vi "OnGameEnd.vi"(8 "error in (no error)":errorcluster, 11 "Game in":refnum<class "Game.lvclass">) -> (0 "error out":errorcluster, 3 "Game out":refnum<class "Game.lvclass">)   [LabVIEW 2019, in "RT_Game.lvlib" / "Game.lvclass"]
uses:
  Game.lvclass
  Game.lvclass/Game.ctl
  Menu/States.ctl
  Highscore/Highscore.lvclass
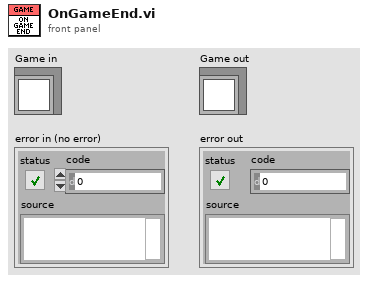
[diagram p1: front panel]
types:
  T1 = typedef "RT_Game.lvlib/Game.lvclass/States.ctl" = enum16{"Init", "Restart", "Menu", "Game", "Resume", "ToggleSingleplayer", "LoadNextGame", "ExitToMenu", "NewHighscore", "GameOver", "SlideOut"}
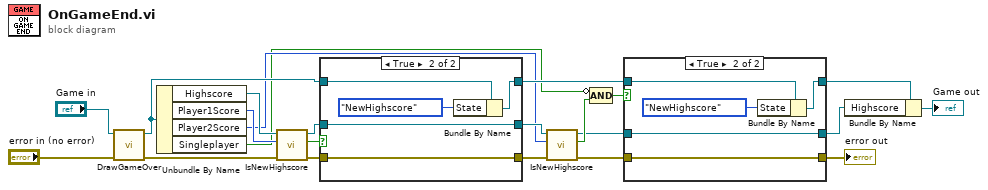
[diagram p0: block diagram]
diagram:
  n1 = call "DrawGameOver.vi"("error in (no error)"="error in (no error)", "Game in"="Game in") -> ("error out"=w20:errorcluster, "Game out"=w13:refnum<class "Game.lvclass">)  [unwired: 8 in]
  n2 = Unbundle By Name(w13) -> ("Highscore"=w18:refnum<class "Highscore.lvclass">, "Player1Score"=w17:i32, "Player2Score"=w6:i32, "Singleplayer"=w1:bool)
  n3 = call "IsNewHighscore.vi"("error in (no error)"=w20, "Score"=w17, "Highscore in"=w18) -> ("error out"=w16:errorcluster, "IsNewHighscore?"=w14:bool, "Highscore out"=w15:refnum<class "Highscore.lvclass">)  [unwired: 6 in]
  n4 = case shown="True" w14 {
    tunnel: w16 -> [w23 w30]
    tunnel: [w23 w30] -> w12
    tunnel: w15 -> [w24 w29]
    tunnel: [w24 w29] -> w11
    tunnel: w13 -> [w25 w28]
    tunnel: [w25 w27] -> w7
    frame False {
    }
    frame True {
      n5 = Bundle By Name(cluster=w28, "State"=States."NewHighscore") -> (w27:refnum<class "Game.lvclass">)
    }
  }
  n6 = call "IsNewHighscore.vi"("error in (no error)"=w12, "Score"=w6, "Highscore in"=w11) -> ("error out"=w3:errorcluster, "IsNewHighscore?"=w5:bool, "Highscore out"=w4:refnum<class "Highscore.lvclass">)  [unwired: 6 in]
  n7 = Compound Arithmetic op=AND(invert w1, w5) -> (w2:bool)
  n8 = case shown="True" w2 {
    tunnel: w3 -> [w31 w38]
    tunnel: [w31 w38] -> w9
    tunnel: w4 -> [w32 w37]
    tunnel: [w32 w37] -> w10
    tunnel: w7 -> [w33 w36]
    tunnel: [w33 w35] -> w8
    frame False {
    }
    frame True {
      n9 = Bundle By Name(cluster=w36, "State"=States."NewHighscore") -> (w35:refnum<class "Game.lvclass">)
    }
  }
  "error out" <- w9
  n10 = Bundle By Name(cluster=w8, "Highscore"=w10) -> (→"Game out":refnum<class "Game.lvclass">)
